vi "ADO Connection Update Data.vi"(5 "condition":string, 7 "data":variant, 8 "error in (no error)":errorcluster caption="错误输入（无错误）", 9 "columns":string[](array[string]), 10 "table":string, 11 "Database Connection 输入":refnum<class "Database Connection.lvclass"> caption="DNL_LabVIEW Object in") -> (0 "error out":errorcluster caption="错误输出", 2 "Database Command 输出":refnum<class "Database Command.lvclass">, 3 "Database Connection 输出":refnum<class "Database Connection.lvclass"> caption="DNL_LabVIEW Object out")   [LabVIEW 2011, in "Database Connection.lvclass"]
uses:
  Database Connection.lvclass
  Command/Database Command.lvclass
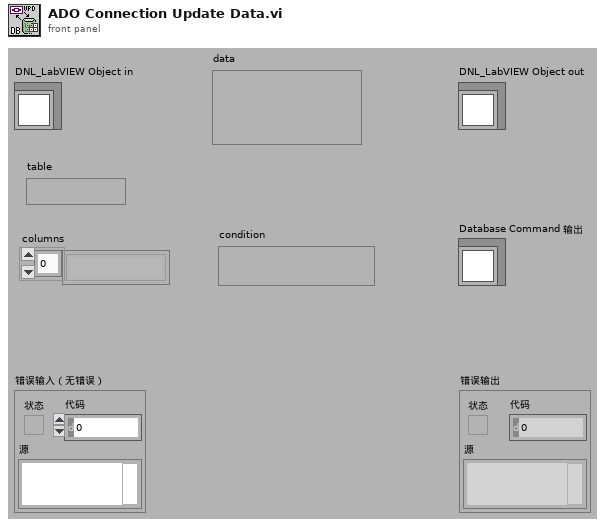
[diagram p1: front panel]
types:
  T1 = typedef "NI_Database_API.lvlib/DB Tools Parameter Info.ctl" = cluster{"parameter name":string, "type":T2, "direction":T3, "value":variant}
  T2 = typedef "NI_Database_API.lvlib/DB Tools DataTypes.ctl" = enum16{"String", "Long (I32)", "Single (SGL)", "Double (DBL)", "Date/Time", "Binary"}
  T3 = typedef "NI_Database_API.lvlib/DB Tools Parameter Dir.ctl" = enum32{"Input", "Output", "Input/Output", "Return Value"}
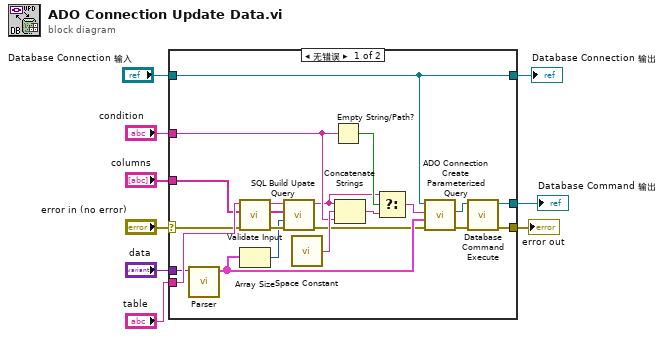
[diagram p0: block diagram]
diagram:
  n1 = case shown="无错误" "error in (no error)" {
    selector: "error in (no error)" -> [w14 w32]
    tunnel: [w11 w32] -> w8
    tunnel: [w23 w31] -> w6
    tunnel: "Database Connection 输入" -> [w23 w31]
    tunnel: "table" -> [w30 _]
    tunnel: "columns" -> [w29 _]
    tunnel: "data" -> [w28 _]
    tunnel: "condition" -> [w19 _]
    tunnel: [w10 _] -> w1
    frame No Error {
      n2 = call "Parser.vi"("variant"=w28) -> ("parameters"=w16:T1[])  [unwired: 9 in, 1 out]
      n3 = call "Validate Input.vi"("error in (no error)"=w14, "columns"=w29, "table"=w30) -> ("error out"=w25:errorcluster, "columns out"=w26:string[], "table out"=w27:string)  [unwired: 6 in]
      n4 = Array Size(array=w16) -> (size(s)=w24:i32)
      n5 = call "SQL Build Upate Query.vi"("error in (no error)"=w25, "num parameters"=w24, "columns"=w26, "table name"=w27) -> ("error out"=w15:errorcluster, "query"=w18:string)  [unwired: 6 in]
      n6 = call <vilib>:"Space Constant.vi"() -> ("String"=w22:string)
      n7 = Empty String/Path?(string/path=w19) -> (empty?=w20:bool)
      n8 = Concatenate Strings(w18, w22, w19) -> (w21:string)
      n9 = Select(t=w18, s=w20, f=w21) -> (s? t:f=w17:string)
      n10 = call "ADO Connection Create Parameterized Query.vi"("error in (no error)"=w15, "parameters"=w16, "SQL query"=w17, "Database Connection 输入"=w23) -> ("error out"=w12:errorcluster, "Database Command 输出"=w13:refnum<class "Database Command.lvclass">)  [unwired: 4 in, 2 out]
      n11 = call "Database Command Execute.vi"("error in (no error)"=w12, "Database Command 输入"=w13) -> ("error out"=w11:errorcluster, "Database Command 输出"=w10:refnum<class "Database Command.lvclass">)  [unwired: 7 in, 1 out]
    }
    frame Error {
    }
  }
  "error out" <- w8
  "Database Connection 输出" <- w6
  "Database Command 输出" <- w1
